vi "execute.vi"(8 "error in (no error)":errorcluster, 9 "image assembler in":refnum<class "GenericComponent.lvclass">, 10 "imaging mode in":refnum<class "GenericComponent.lvclass">, 11 "DL090309ImagingModeToImageAssemblerAdapter in":refnum<class "AdapterDL090309ImagingModeToImageAssembler.lvclass">) -> (0 "error out":errorcluster, 1 "image assembler out":refnum<class "GenericComponent.lvclass">, 2 "imaging mode out":refnum<class "GenericComponent.lvclass">, 3 "DL090309ImagingModeToImageAssemblerAdapter out":refnum<class "AdapterDL090309ImagingModeToImageAssembler.lvclass">)   [LabVIEW 2010, in "AdapterDL090309ImagingModeToImageAssembler.lvclass"]
uses:
  AdapterDL090309ImagingModeToImageAssembler.lvclass
  common/classes/GenericComponent/GenericComponent/GenericComponent.lvclass
  ImageAssembler/ImageAssemblerDL090211Frame/ImageAssemblerDL090211Frame/ImageAssemblerDL090211Frame.lvclass
  ImagingMode/ImagingModeDL090130Frame/ImagingModeDL090130Frame/ImagingModeDL090130Frame.lvclass
  ImageAssembler/ImageAssemblerDL090211Scaffold/ImageAssemblerDL090211Scaffold/ImageAssemblerDL090211Scaffold.lvclass
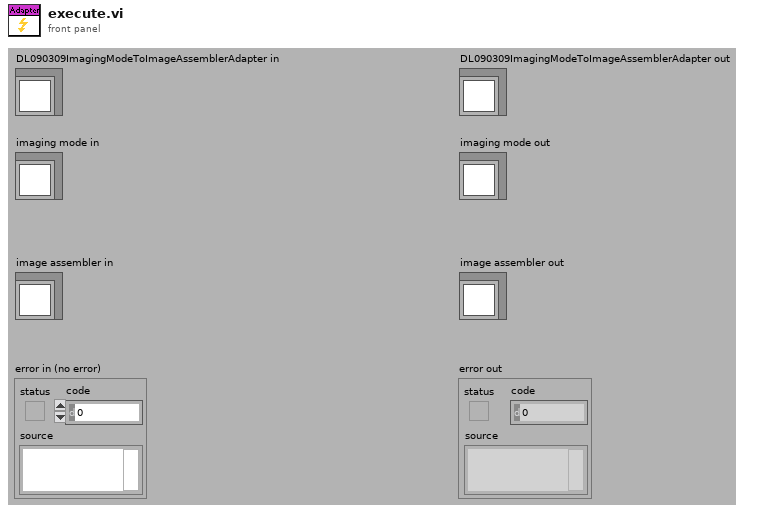
[diagram p1: front panel]
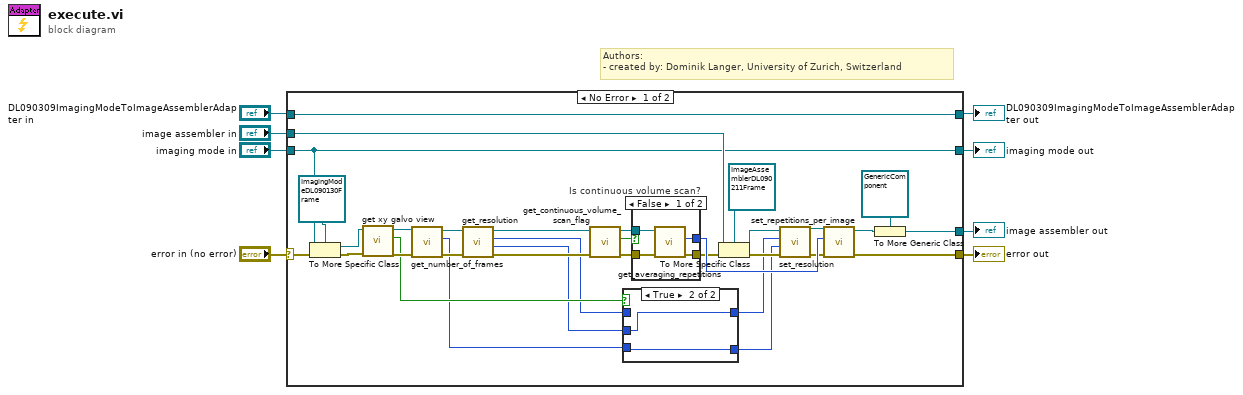
[diagram p0: block diagram]
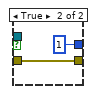
[diagram p3: hidden frame]
diagram:
  # "Authors: \n- created by: Dominik Langer, University of Zurich, Switzerland"
  n1 = case shown="No Error" "error in (no error)" {
    selector: "error in (no error)" -> [w33 w55]
    tunnel: [w27 w55] -> w7
    tunnel: [w31 w54] -> w5
    tunnel: "DL090309ImagingModeToImageAssemblerAdapter in" -> [w31 w54]
    tunnel: "imaging mode in" -> [w29 w52]
    tunnel: "image assembler in" -> [w32 w53]
    tunnel: [w30 w53] -> w2
    tunnel: [w29 w52] -> w1
    frame No Error {
      n2 = To More Specific Class(target class=refnum<class "ImagingModeDL090130Frame.lvclass"> refnum ("DL090130FrameScanMode.lvclass"), reference=w29, error in=w33) -> (specific class reference=w17:refnum<class "ImagingModeDL090130Frame.lvclass">, error out=w18:errorcluster)
      n3 = call-dynamic "get xy galvo view.vi"("error in (no error)"=w18, "ImagingModeDL090130Frame in"=w17) -> ("error out"=w15:errorcluster, "xy galvo view?"=w14:bool, "ImagingModeDL090130Frame out"=w16:refnum<class "ImagingModeDL090130Frame.lvclass">)  [unwired: 7 in]
      n4 = call-dynamic "get_number_of_frames.vi"("error in (no error)"=w15, "ImagingModeDL090130Frame in"=w16) -> ("error out"=w19:errorcluster, "number of frames"=w9:i32, "ImagingModeDL090130Frame out"=w20:refnum<class "ImagingModeDL090130Frame.lvclass">)  [unwired: 7 in]
      n5 = call-dynamic "get_resolution.vi"("error in (no error)"=w19, "ImagingModeDL090130Frame in"=w20) -> ("error out"=w25:errorcluster, "y resolution"=w13:i32, "x resolution"=w10:i32, "ImagingModeDL090130Frame out"=w22:refnum<class "ImagingModeDL090130Frame.lvclass">)  [unwired: 6 out]
      n6 = call "get_continuous_volume_scan_flag.vi"("error in (no error)"=w25, "ImagingModeDL090130Frame in"=w22) -> ("error out"=w24:errorcluster, "is continuous volume scan?"=w23:bool, "ImagingModeDL090130Frame out"=w21:refnum<class "ImagingModeDL090130Frame.lvclass">)  [unwired: 7 in]
      n7 = case shown="True" w14 {
        tunnel: [w43 w44] -> w12
        tunnel: w13 -> [w43 w45]
        tunnel: w10 -> [w42 _]
        tunnel: [w42 w45] -> w11
        tunnel: w9 -> [_ w44]
        frame False {
        }
        frame True {
        }
      }
      n8 = case "Is continuous volume scan?" shown="False" w23 {
        tunnel: [w49 1 ("averaging repetitions")] -> w36
        tunnel: [w48 w50] -> w26
        tunnel: w21 -> [w47 _]
        tunnel: w24 -> [w46 w50]
        frame False {
          n9 = call-dynamic "get_averaging_repetitions.vi"("error in (no error)"=w46, "ImagingModeDL090130Frame in"=w47) -> ("error out"=w48:errorcluster, "averaging repetitions"=w49:i32)  [unwired: 8 out]
        }
        frame True {
        }
      }
      n10 = To More Specific Class(target class=refnum<class "ImageAssemblerDL090211Frame.lvclass"> refnum ("DL090211FrameImageAssembler.lvclass"), reference=w32, error in=w26) -> (specific class reference=w38:refnum<class "ImageAssemblerDL090211Frame.lvclass">, error out=w37:errorcluster)
      n11 = call "set_resolution.vi"("error in (no error)"=w37, "y resolution"=w12, "x resolution"=w11, "DL090211FrameImageAssembler.lvclass in"=w38) -> ("error out"=w35:errorcluster, "DL090211FrameImageAssembler.lvclass out"=w41:refnum<class "ImageAssemblerDL090211Frame.lvclass">)  [unwired: 6 out]
      n12 = call "set_repetitions_per_image.vi"("error in (no error)"=w35, "repetitions per image"=w36, "DL090211ImageAssemblerScaffold.lvclass in"=w41) -> ("error out"=w27:errorcluster, "DL090211ImageAssemblerScaffold.lvclass out"=w28:refnum<class "ImageAssemblerDL090211Frame.lvclass">)  [unwired: 7 out]
      n13 = To More Generic Class(target class=refnum<class "GenericComponent.lvclass"> refnum ("GenericComponent.lvclass"), reference=w28) -> (generic class reference=w30:refnum<class "GenericComponent.lvclass">)
    }
    frame Error {
    }
  }
  "error out" <- w7
  "DL090309ImagingModeToImageAssemblerAdapter out" <- w5
  "image assembler out" <- w2
  "imaging mode out" <- w1
